vi "Actor Core.vi"(8 "error in":errorcluster, 11 "QuadLayout in":refnum<class "QuadViewManager.lvclass">=refnum) -> (0 "error out":errorcluster, 3 "Actor out":refnum<class "Actor.lvclass">)   [LabVIEW 2015, in "QuadViewManager.lvlib" / "QuadViewManager.lvclass"]
doc: "(<B>Filename</B>: Actor Framework.lvlib:Actor.lvclass:Actor Core.vi)\n\nReceives messages to the actor, reacts to them, and initiates any error handling that may shut the actor down.\n\nDescendant classes may override this VI to append parallel tasks for the actor to complete while it handles messages. Overrides use the Call Parent Method node.\n\n<License>\nCopyright © 2017 Composed Systems, LLC | All rights reserved\nwww.composed.io\n\nAuthor: Ethan Stern <ethan.stern@composed.io>\n\nThis software is provided \"AS IS\" WITHOUT WARRANTIES, either express or implied, AND IS FOR EDUCATIONAL PURPOSES ONLY.\n</License>"
uses:
  QuadViewManager.lvclass
  <vilib>/ActorFramework/Actor/Actor.lvclass
  QuadViewManager.lvclass/QuadViewManager.ctl
  Framework/IViewManager/IViewManager/IViewManager.lvclass
  Framework/Components/ProtectedSubpanel/ProtectedSubpanel.lvclass
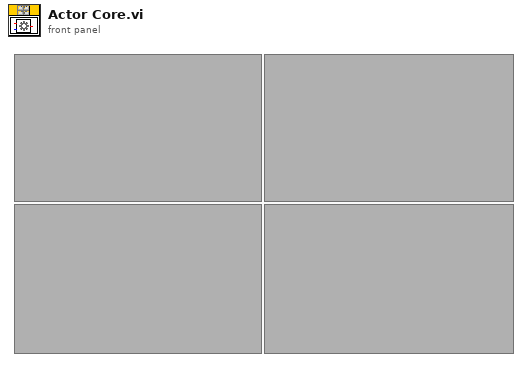
[diagram p1: front panel]
types:
  T1 = typedef "ProtectedSubpanel.lvlib/ProtectedSubpanel.lvclass/Protected Subpanel Reference.ctl" = refnum<data-value>
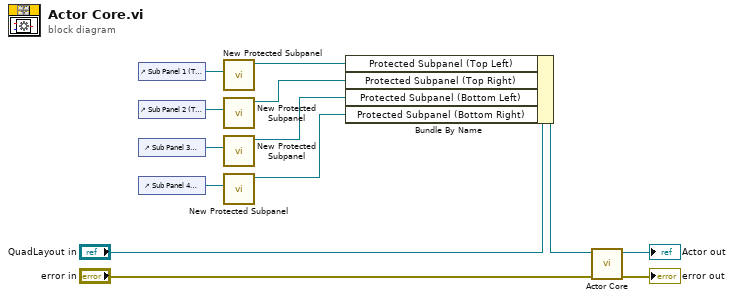
[diagram p0: block diagram]
diagram:
  n1 = control-ref of="Sub Panel 1 (Top Left)"() -> (w8:refnum<vi>)
  n2 = control-ref of="Sub Panel 2 (Top Right)"() -> (w6:refnum<vi>)
  n3 = control-ref of="Sub Panel 3 (Bottom Left)"() -> (w5:refnum<vi>)
  n4 = control-ref of="Sub Panel 4 (Bottom Right)"() -> (w4:refnum<vi>)
  n5 = call "New Protected Subpanel.vi"("SubPnl Refnum"=w8) -> ("Protected Subpanel"=w7:T1)  [unwired: 9 in, 1 out]
  n6 = call "New Protected Subpanel.vi"("SubPnl Refnum"=w6) -> ("Protected Subpanel"=w1:T1)  [unwired: 9 in, 1 out]
  n7 = call "New Protected Subpanel.vi"("SubPnl Refnum"=w5) -> ("Protected Subpanel"=w2:T1)  [unwired: 9 in, 1 out]
  n8 = call "New Protected Subpanel.vi"("SubPnl Refnum"=w4) -> ("Protected Subpanel"=w3:T1)  [unwired: 9 in, 1 out]
  n9 = Bundle By Name(cluster="QuadLayout in", "Protected Subpanel (Top Left)"=w7, "Protected Subpanel (Top Right)"=w1, "Protected Subpanel (Bottom Left)"=w2, "Protected Subpanel (Bottom Right)"=w3) -> (w9:refnum<class "QuadViewManager.lvclass">)
  n10 = call-parent "Actor Core.vi"("error in"="error in", "IViewable In"=w9) -> ("error out"=→"error out":errorcluster, "Actor out"=→"Actor out":refnum<class "Actor.lvclass">)  [unwired: 8 in]
